vi "Test Classes 2.vi"() -> ()   [LabVIEW 2009]
uses:
  LV-BME Interface/ChnlSettings.ctl
  LV-BME Interface/BME_DG_TriggerSettings.ctl
  LV-BME Interface/ClockSource.ctl
  DG Classes/BME_DG_G08/G08TriggerSettings.ctl
  DG Classes/BME_DG_System/BME_DG_System.lvclass
  DG Classes/BME_DG_G08/BME_DG_G08.lvclass
  DG Classes/BME_DG_G08_Chnl/BME_DG_G08_Chnl.lvclass
  DG Classes/BME_DG_Base/BME_DG_Base.lvclass
  DG Classes/BME_DG_Chnl/BME_DG_Chnl.lvclass
panel:
  in  "Aknowledge interrupts":bool
  in  "stop 3":bool=TRUE
  in  "G08Settings":T1={"Gate Terminate"=TRUE, "Gate Level"=1.0, "Gate Delay (µs)"=0.0, "Step Back Time (µs)"=0.0, "Burst Counter"=0} {"Step Back Time (µs)" min=0.0 format="%.6f"; "Gate Delay (µs)" format="%.3f"; "Gate Level" min=-2.5 max=2.5 format="%.3g"}
  in  "V2 Trigger Settings":T2={"Gate Type"=TRUE, "Synchronize Gate"=FALSE, "Force Trigger (µs)"=0.0, "MS Bus"=1} {"MS Bus" format="%04x" items=["Local Primary"=1, "Local Secondary"=2, "Local Force"=4, "Resynchronize"=8, "Master Primary"=16, "Master Secondary"=32, "Master Force"=64, "System Clock"=128, "Delay Clock"=256, "Inhibit Local"=512, "Start Local"=1024, "Start Bus"=2048, "Step Back Local"=4096, "Step Back Bus"=8192, "Enable From E"=65536, "Enable From F"=131072, "Enable From Bus"=262144]; "Force Trigger (µs)" min=0.0 format="%.6f"}
  in  "SetDelay":bool=TRUE
  in  "UpdateChnl":bool=TRUE
  in  "ChnlParameter":T4 {"ChnParam2write"."Delay (µs)" min=0.0 max=100000000.0 format="%.5f"}
  out "CountsRemains":i32
  out "TriggerCounters":i32[](array[numeric])
  out "Interrupts":u32[](array[numeric]) format="%b"
  in  "ClockSource Master":T5=1 items=["Internal Oscillator"=1, "External Trigger"=2, "Trigger & Oscillator"=3, "MasterSlave Bus"=4]
  in  "Trigger Settings SG02P2":T6={"InputTerminated?"=FALSE, "InternalClockPeriode(µs)"=1000000.0, "TriggerLevel"=1.25, "PresetValue"=0, "DivideBy"=1, "Clock Source"=1, "Gate Divider"=1, "PositiveGate?"=TRUE, "InternalTrigger?"=TRUE, "InternalArm?"=FALSE, "SWTrigger?"=FALSE, "RisingEdge?"=FALSE, "StopOnPreset?"=FALSE, "ResetWhenDone?"=TRUE, "TriggerEnabled?"=TRUE} {"Gate Divider" min=1 max=1000000; "Clock Source" items=["Internal Oscillator"=1, "External Trigger"=2, "Trigger & Oscillator"=3]}
  out "RemainingTriggers":T7(array[cluster])=[[{"Time Stamp"=timestamp(3416308194.6875 s since 1904-01-01), "Numeric"=-64}, {"Time Stamp"=timestamp(3416308194.6875 s since 1904-01-01), "Numeric"=4}, {"Time Stamp"=timestamp(3416308194.6875 s since 1904-01-01), "Numeric"=-64}, {"Time Stamp"=timestamp(3416308194.6875 s since 1904-01-01), "Numeric"=-64}], [{"Time Stamp"=timestamp(3416308194.6875 s since 1904-01-01), "Numeric"=-64}, {"Time Stamp"=timestamp(3416308194.6875 s since 1904-01-01), "Numeric"=-64}, {"Time Stamp"=timestamp(3416308194.6875 s since 1904-01-01), "Numeric"=-64}, {"Time Stamp"=timestamp(3416308194.6875 s since 1904-01-01), "Numeric"=-64}], [{"Time Stamp"=timestamp(3416308194.6875 s since 1904-01-01), "Numeric"=-64}, {"Time Stamp"=timestamp(3416308194.6875 s since 1904-01-01), "Numeric"=-64}, {"Time Stamp"=timestamp(3416308194.6875 s since 1904-01-01), "Numeric"=-64}, {"Time Stamp"=timestamp(3416308194.6875 s since 1904-01-01), "Numeric"=-64}]] {"Time Stamp" format="%<%I:%M:%S%3u %p>T"}
  in  "stop 2":bool=TRUE
  in  "ReadStatus":bool=TRUE
  in  "Activate":bool
  in  "ResetModuloCounters":bool=TRUE
  in  "TriggerModulo":u32=4
  out "Modulo Settings":u32[](array[numeric])
  out "Chnls":T3[](array[typedef])=[{" Delay (µs)"=0.0, "On? (false)"=TRUE, "PositiveVoltage?"=TRUE, "50OhmTerminated? "=TRUE, "25OhmOutput?"=FALSE}, {" Delay (µs)"=0.0, "On? (false)"=TRUE, "PositiveVoltage?"=TRUE, "50OhmTerminated? "=TRUE, "25OhmOutput?"=FALSE}, {" Delay (µs)"=0.0, "On? (false)"=TRUE, "PositiveVoltage?"=TRUE, "50OhmTerminated? "=TRUE, "25OhmOutput?"=FALSE}] {"Delay (µs)" min=0.0 max=100000000.0 format="%.5f"}
  in  "Trigger Base":T6={"InputTerminated?"=FALSE, "InternalClockPeriode(µs)"=1000000.0, "TriggerLevel"=1.25, "PresetValue"=0, "DivideBy"=1, "Clock Source"=1, "Gate Divider"=1, "PositiveGate?"=TRUE, "InternalTrigger?"=FALSE, "InternalArm?"=FALSE, "SWTrigger?"=FALSE, "RisingEdge?"=FALSE, "StopOnPreset?"=FALSE, "ResetWhenDone?"=TRUE, "TriggerEnabled?"=TRUE} {"Gate Divider" min=1 max=1000000; "Clock Source" items=["Internal Oscillator"=1, "External Trigger"=2, "Trigger & Oscillator"=3]}
  in  "Selected Chnl":u16(ring) items=["MasterS08P1_ChnlA", "MasterS08P1_ChnlB", "MasterS08P1_ChnlC", "MasterS08P1_ChnlD", "MasterS08P1_ChnlE", "MasterS08P1_ChnlF"]
  in  "Selected Card":u16(ring)=1 items=["MasterSG02P2", "Slave 1", "Slave 2", "MasterS08P1"]
  in  "STOP":bool=TRUE
  in  "ChnParam2write":T3={" Delay (µs)"=0.0, "On? (false)"=TRUE, "PositiveVoltage?"=TRUE, "50OhmTerminated? "=TRUE, "25OhmOutput?"=FALSE} {"Delay (µs)" min=0.0 max=100000000.0 format="%.5f"}
  # "INIT Values"
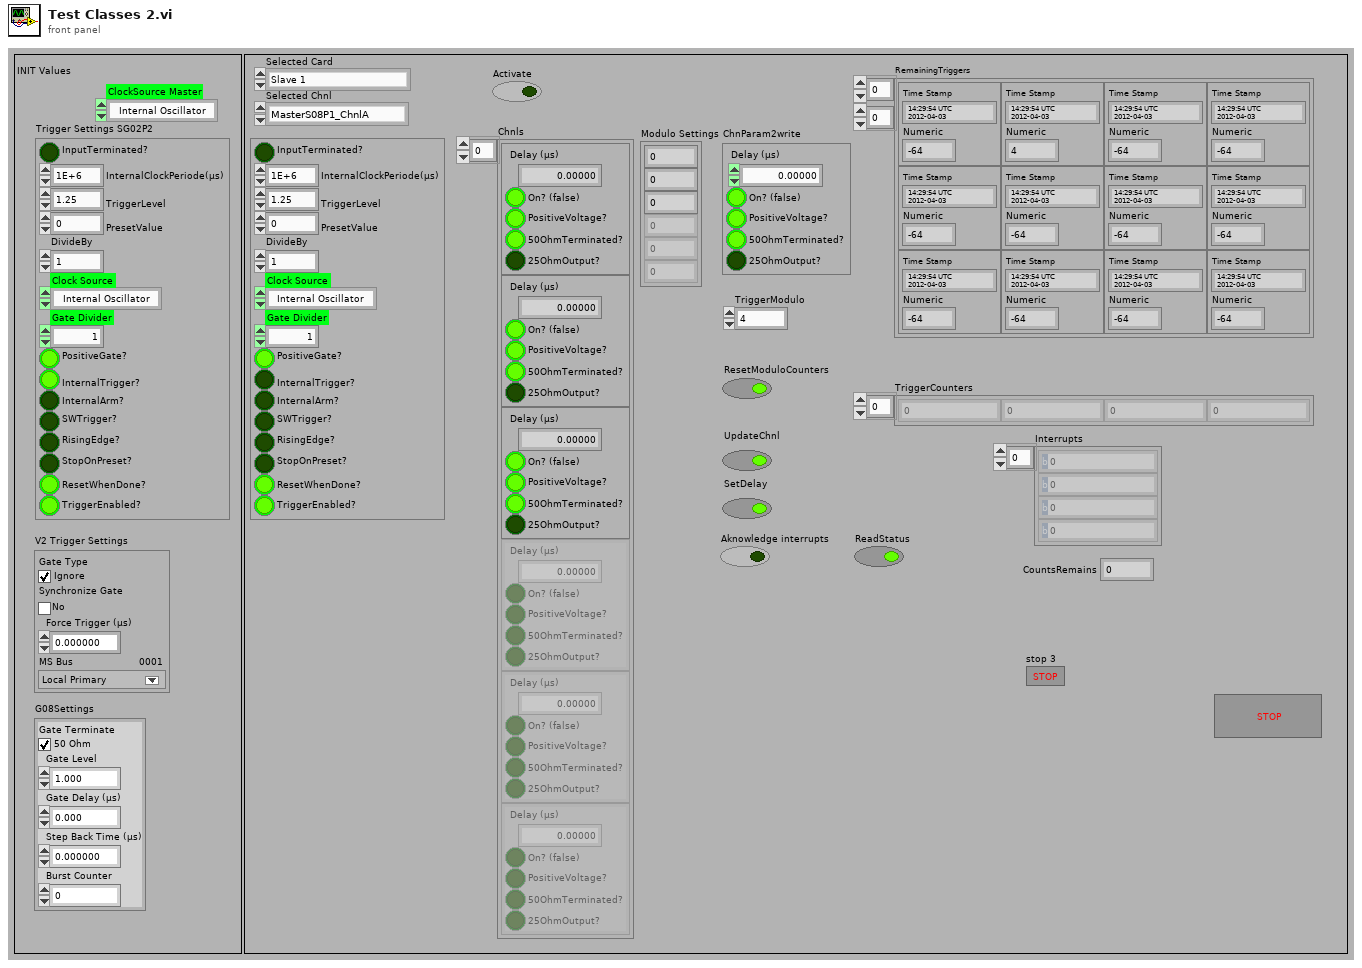
[diagram p1: front panel]
types:
  T1 = typedef "BME_DG_G08.lvclass/G08TriggerSettings.ctl" = cluster{"Gate Terminate":bool, "Gate Level":dbl, "Gate Delay (µs)":dbl, "Step Back Time (µs)":dbl, "Burst Counter":u32}
  T2 = cluster{"Gate Type":bool, "Synchronize Gate":bool, "Force Trigger (µs)":dbl, "MS Bus":u32}
  T3 = typedef "ChnlSettings.ctl" = cluster{" Delay (µs)":dbl, "On? (false)":bool, "PositiveVoltage?":bool, "50OhmTerminated? ":bool, "25OhmOutput?":bool}
  T4 = cluster{"ChnlName":string, "ChnParam2write":T3, "TriggerModulo":u32}
  T5 = typedef "ClockSource.ctl" = i32
  T6 = typedef "BME_DG_TriggerSettings.ctl" = cluster{"InputTerminated?":bool, "InternalClockPeriode(µs)":dbl, "TriggerLevel":dbl, "PresetValue":i32, "DivideBy":i32, "Clock Source":u32, "Gate Divider":i32, "PositiveGate?":bool, "InternalTrigger?":bool, "InternalArm?":bool, "SWTrigger?":bool, "RisingEdge?":bool, "StopOnPreset?":bool, "ResetWhenDone?":bool, "TriggerEnabled?":bool}
  T7 = cluster{"Time Stamp":timestamp, "Numeric":i32}[][]
  T8 = enum8{"Enabled", "Disabled", "Disabled and Grayed Out"}
  T9 = cluster{"ChnlName":string, "ChnParam2write":T3, "TriggerModulo":u32}[]
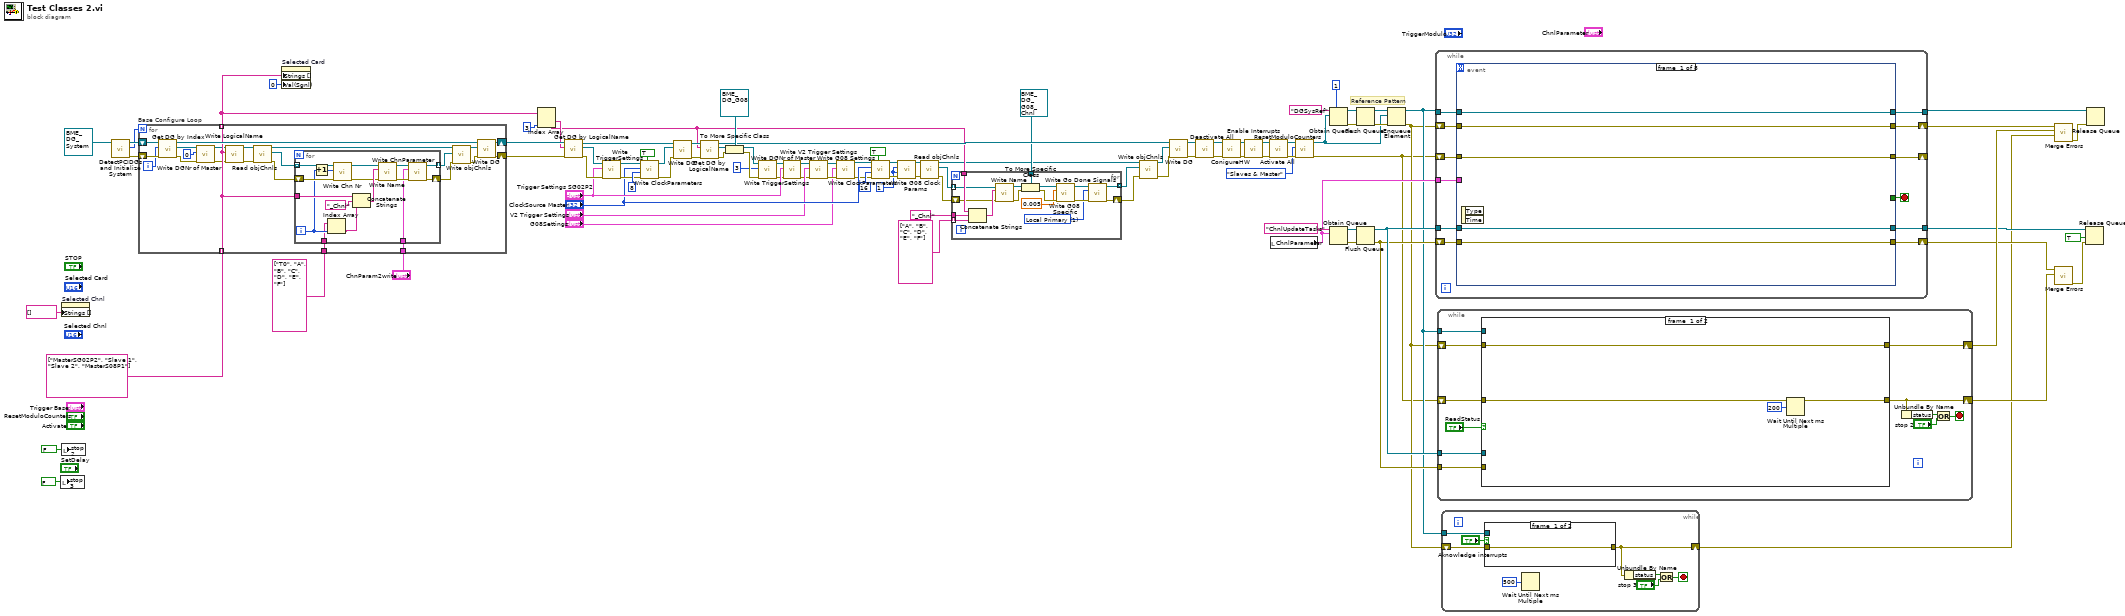
[diagram p0: block diagram]
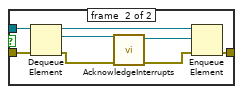
[diagram p2: hidden frame]
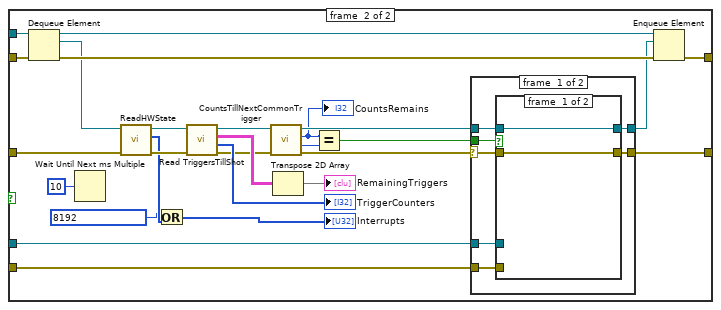
[diagram p3: hidden frame]
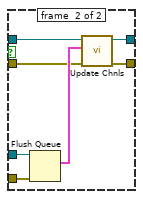
[diagram p4: hidden frame]
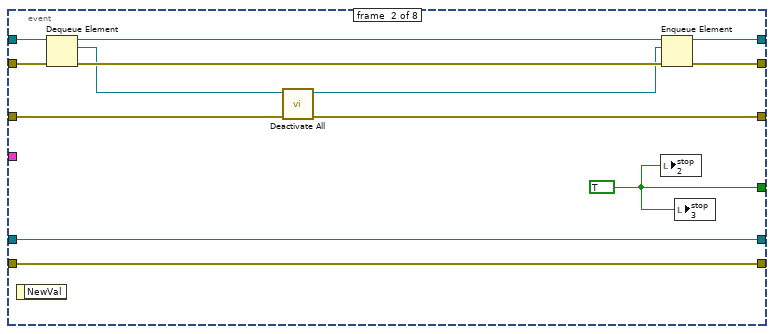
[diagram p6: hidden frame]
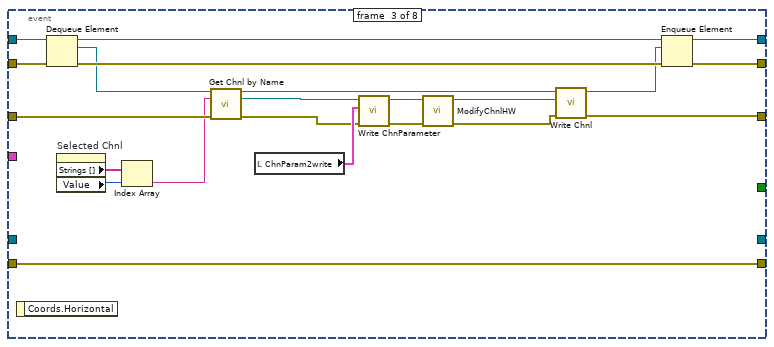
[diagram p7: hidden frame]
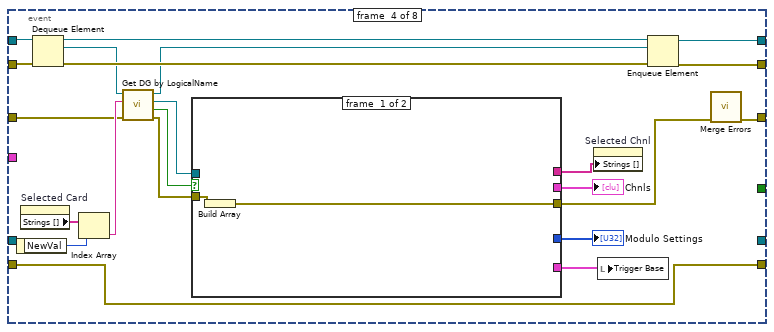
[diagram p8: hidden frame]
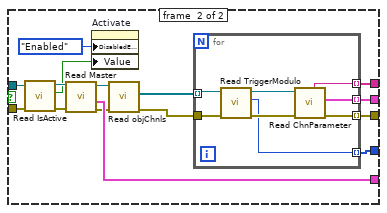
[diagram p9: hidden frame]
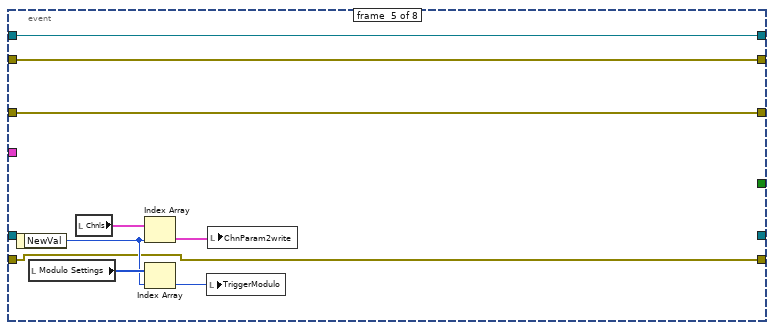
[diagram p10: hidden frame]
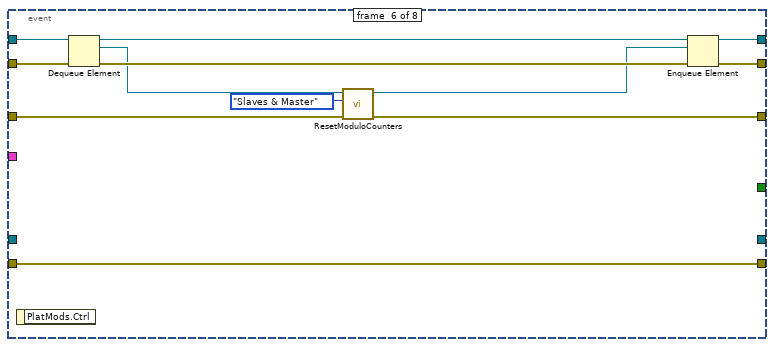
[diagram p11: hidden frame]
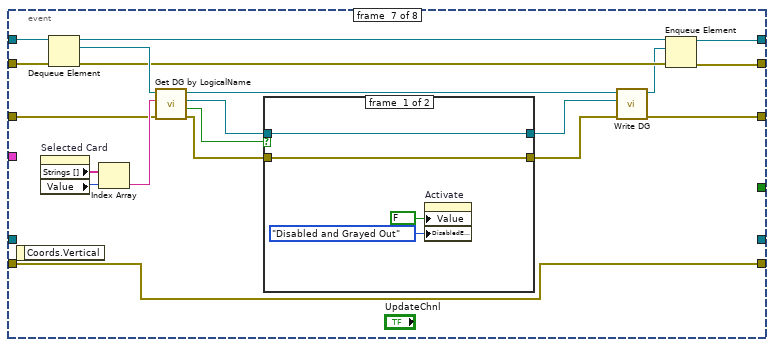
[diagram p12: hidden frame]
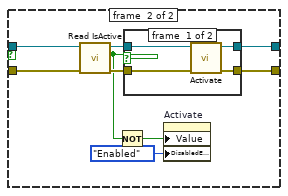
[diagram p13: hidden frame]
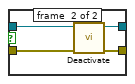
[diagram p14: hidden frame]
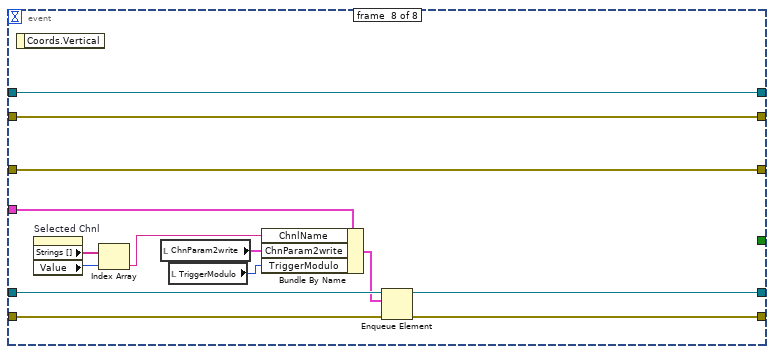
[diagram p15: hidden frame]
diagram:
  w35 = u32 1 ("Trigger Divider")
  # "Reference Pattern"
  n1 = local write "stop 3"(FALSE ("stop 3")) -> ()
  n2 = property on="Selected Chnl" class="Ring (strict)"("Strings []"=string[] []) -> ()  [unwired: 2 in, 2 out]
  n3 = local write "stop 2"(FALSE ("stop 2")) -> ()
  n4 = call "DetectPCIDGs and Initialize System.vi"("BME_DG_System in"=refnum<class "BME_DG_System.lvclass"> refnum ("BME_DG_System.lvclass")) -> ("error out"=w99:errorcluster, "NumberOfCards"=w98:i32, "BME_DG_System out"=w100:refnum<class "BME_DG_System.lvclass">)  [unwired: 8 in]
  n5 = for "Base Configure Loop" {
    N: w98 -> [_]
    shift-right: [w120] -> w68
    shift-left: w100 -> [w124]
    tunnel: string[] ["MasterSG02P2", "Slave 1", "Slave 2", "MasterS08P1"] -> [w109] mode=indexing
    shift-right: [w119] -> w67
    shift-left: w99 -> [w123]
    tunnel: "ChnParam2write" -> [w116]
    tunnel: string[] ["T0", "A", "B", "C", "D", "E", "F"] -> [w110]
    tunnel: [w109] -> w66 mode=indexing
    i -> [w122]
    n6 = call "Get DG by Index.vi"("error in (no error)"=w123, "index"=w122, "BME_DG_System in"=w124) -> ("error out"=w103:errorcluster, "BME_DG_Base.lvclass"=w106:refnum<class "BME_DG_Base.lvclass">, "BME_DG_System out"=w121:refnum<class "BME_DG_System.lvclass">)  [unwired: 6 in]
    n7 = call-dynamic "Write DGNr of Master.vi"("error in (no error)"=w103, "DGNr of Master"=0, "BME_DG_Base in"=w106) -> ("error out"=w104:errorcluster, "BME_DG_Base out"=w105:refnum<class "BME_DG_Base.lvclass">)  [unwired: 7 in]
    n8 = call "Write LogicalName.vi"("error in (no error)"=w104, "LogicalName"=w109, "BME_DG_Base in"=w105) -> ("error out"=w107:errorcluster, "BME_DG_Base out"=w108:refnum<class "BME_DG_Base.lvclass">)  [unwired: 7 in]
    n9 = call-dynamic "Read objChnls.vi"("error in (no error)"=w107, "BME_DG_Base in"=w108) -> ("error out"=w117:errorcluster, "objChnls"=w118:refnum<class "BME_DG_Chnl.lvclass">[], "BME_DG_Base out"=w114:refnum<class "BME_DG_Base.lvclass">)  [unwired: 6 in, 1 out]
    n10 = for {
      tunnel: w118 -> [w134] mode=indexing
      shift-right: [w125] -> w112
      shift-left: w117 -> [w132]
      tunnel: w109 -> [w139]
      tunnel: w116 -> [w135]
      tunnel: [w126] -> w115 mode=indexing
      tunnel: w110 -> [w128]
      i -> [w129]
      n11 = Increment(x=w129) -> (x+1=w130:i32)
      n12 = Index Array(array=w128, index=w129) -> (element=w127:string)
      n13 = call-dynamic "Write Chn Nr.vi"("error in (no error)"=w132, "Chn Nr"=w130, "BME_DG_Chnl in"=w134) -> ("error out"=w131:errorcluster, "BME_DG_Chnl out"=w133:refnum<class "BME_DG_Chnl.lvclass">)  [unwired: 7 in]
      n14 = Concatenate Strings(w139, "_Chnl" ("string"), w127) -> (w137:string)
      n15 = call-dynamic "Write Name.vi"("error in (no error)"=w131, "Name"=w137, "BME_DG_Chnl in"=w133) -> ("error out"=w136:errorcluster, "BME_DG_Chnl out"=w140:refnum<class "BME_DG_Chnl.lvclass">)  [unwired: 7 in]
      n16 = call-dynamic "Write ChnParameter.vi"("error in (no error)"=w136, "ChnParemater"=w135, "BME_DG_Chnl in"=w140) -> ("error out"=w125:errorcluster, "BME_DG_Chnl out"=w126:refnum<class "BME_DG_Chnl.lvclass">)  [unwired: 7 in]
    }
    n17 = call-dynamic "Write objChnls.vi"("error in (no error)"=w112, "objChnls"=w115, "BME_DG_Base in"=w114) -> ("error out"=w111:errorcluster, "BME_DG_Base out"=w113:refnum<class "BME_DG_Base.lvclass">)  [unwired: 7 in]
    n18 = call "Write DG.vi"("error in (no error)"=w111, "BME_DG_Base"=w113, "BME_DG_System in"=w121) -> ("error out"=w119:errorcluster, "BME_DG_System out"=w120:refnum<class "BME_DG_System.lvclass">)  [unwired: 7 in]
  }
  n19 = property on="Selected Card" class="Ring (strict)"("Strings []"=w66, "Val(Sgnl)"=u16 0 ("Value (Signaling)")) -> ()  [unwired: 2 in, 2 out]
  n20 = Index Array(array=w66, index #2=3 ("index")) -> (element #1=w64:string, element #2=w30:string)  [unwired: 1 in]
  n21 = call "Get DG by LogicalName.vi"("error in (no error)"=w67, "LogicalName"=w64, "BME_DG_System in"=w68) -> ("error out"=w62:errorcluster, "BME_DG_Base.lvclass"=w63:refnum<class "BME_DG_Base.lvclass">, "BME_DG_System out"=w59:refnum<class "BME_DG_System.lvclass">)  [unwired: 5 in, 1 out]
  n22 = call-dynamic "Write TriggerSettings.vi"("error in (no error)"=w62, "Trigger Settings"="Trigger Settings SG02P2", "BME_DG_Base in"=w63) -> ("error out"=w60:errorcluster, "BME_DG_Base out"=w61:refnum<class "BME_DG_Base.lvclass">)  [unwired: 7 in]
  n23 = call-dynamic "Write ClockParameters.vi"("ClockEnable"=TRUE, "error in (no error)"=w60, "PrescalerCrystalOscilator"=u32 8 ("DivideBy"), "ClockSource"="ClockSource Master", "BME_DG_Base in"=w61) -> ("error out"=w57:errorcluster, "BME_DG_Base out"=w58:refnum<class "BME_DG_Base.lvclass">)  [unwired: 5 in]
  n24 = call "Write DG.vi"("error in (no error)"=w57, "BME_DG_Base"=w58, "BME_DG_System in"=w59) -> ("error out"=w56:errorcluster, "BME_DG_System out"=w55:refnum<class "BME_DG_System.lvclass">)  [unwired: 7 in]
  n25 = call "Get DG by LogicalName.vi"("error in (no error)"=w56, "LogicalName"=w30, "BME_DG_System in"=w55) -> ("error out"=w45:errorcluster, "BME_DG_Base.lvclass"=w50:refnum<class "BME_DG_Base.lvclass">, "BME_DG_System out"=w41:refnum<class "BME_DG_System.lvclass">)  [unwired: 5 in, 1 out]
  n26 = To More Specific Class(target class=refnum<class "BME_DG_G08.lvclass"> refnum ("BME_DG_G08.lvclass"), reference=w50, error in=w45) -> (specific class reference=w16:refnum<class "BME_DG_G08.lvclass">, error out=w14:errorcluster)
  n27 = call-dynamic "Write DGNr of Master.vi"("error in (no error)"=w14, "DGNr of Master"=3, "BME_DG_Base in"=w16) -> ("error out"=w13:errorcluster, "BME_DG_Base out"=w15:refnum<class "BME_DG_G08.lvclass">)  [unwired: 7 in]
  n28 = call-dynamic "Write TriggerSettings.vi"("error in (no error)"=w13, "Trigger Settings"="Trigger Settings SG02P2", "BME_DG_Base in"=w15) -> ("error out"=w46:errorcluster, "BME_DG_Base out"=w48:refnum<class "BME_DG_G08.lvclass">)  [unwired: 7 in]
  n29 = call-dynamic "Write V2 Trigger Settings.vi"("error in (no error)"=w46, "V2 Trigger Settings"="V2 Trigger Settings", "BME_DG_G05 in"=w48) -> ("error out"=w43:errorcluster, "BME_DG_G05 out"=w44:refnum<class "BME_DG_G08.lvclass">)  [unwired: 7 in]
  n30 = call-dynamic "Write G08 Settings.vi"("error in (no error)"=w43, "G08Settings"="G08Settings", "BME_DG_G08 in"=w44) -> ("error out"=w38:errorcluster, "BME_DG_G08 out"=w39:refnum<class "BME_DG_G08.lvclass">)  [unwired: 7 in]
  n31 = call-dynamic "Write ClockParameters.vi"("ClockEnable"=TRUE, "error in (no error)"=w38, "PrescalerCrystalOscilator"=u32 16, "ClockSource"="ClockSource Master", "BME_DG_Base in"=w39) -> ("error out"=w36:errorcluster, "BME_DG_Base out"=w37:refnum<class "BME_DG_G08.lvclass">)  [unwired: 5 in]
  n32 = call-dynamic "Write G08 Clock Params.vi"("error in (no error)"=w36, "Trigger Multiplier"=w35, "Trigger Divider"=w35, "BME_DG_G08 in"=w37) -> ("error out"=w33:errorcluster, "BME_DG_G08 out"=w34:refnum<class "BME_DG_G08.lvclass">)  [unwired: 6 in]
  n33 = call-dynamic "Read objChnls.vi"("error in (no error)"=w33, "BME_DG_Base in"=w34) -> ("error out"=w29:errorcluster, "objChnls"=w32:refnum<class "BME_DG_Chnl.lvclass">[], "BME_DG_Base out"=w25:refnum<class "BME_DG_G08.lvclass">)  [unwired: 6 in, 1 out]
  n34 = for {
    tunnel: w32 -> [w155] mode=indexing
    tunnel: string[] ["A", "B", "C", "D", "E", "F"] -> [w157] mode=indexing
    tunnel: w30 -> [w156]
    shift-right: [w144] -> w26
    shift-left: w29 -> [w153]
    tunnel: "_Chnl" ("string") -> [w152]
    tunnel: refnum<class "BME_DG_G08_Chnl.lvclass"> refnum ("BME_DG_G08_Chnl.lvclass") -> [w149]
    tunnel: [w142] -> w24 mode=indexing
    w143 = u32 1 items=["Local Primary"=1, "Local Secondary"=2, "Local Force"=4, "Resynchronize"=8, "Master Primary"=16, "Master Secondary"=32, "Master Force"=64, "System Clock"=128, "Delay Clock"=256, "Inhibit Local"=512, "Start Local"=1024, "Start Bus"=2048, "Step Back Local"=4096, "Step Back Bus"=8192, "From E"=65536, "From F"=131072, "From Bus"=262144] ("Go Signal")
    n35 = Concatenate Strings(w156, w152, w157) -> (w154:string)
    n36 = call-dynamic "Write Name.vi"("error in (no error)"=w153, "Name"=w154, "BME_DG_Chnl in"=w155) -> ("error out"=w148:errorcluster, "BME_DG_Chnl out"=w151:refnum<class "BME_DG_Chnl.lvclass">)  [unwired: 7 in]
    n37 = To More Specific Class(target class=w149, reference=w151, error in=w148) -> (specific class reference=w150:refnum<class "BME_DG_G08_Chnl.lvclass">, error out=w147:errorcluster)
    n38 = call-dynamic "Write G08 Specific.vi"("error in (no error)"=w147, "Pulse Width (µs)"=0.005, "BME_DG_G08_Chnl in"=w150) -> ("error out"=w145:errorcluster, "BME_DG_G08_Chnl out"=w146:refnum<class "BME_DG_G08_Chnl.lvclass">)  [unwired: 7 in]
    n39 = call-dynamic "Write Go Done Signals.vi"("error in (no error)"=w145, "Go Signal"=w143, "BME_DG_G05P2_Chnl in"=w146) -> ("error out"=w144:errorcluster, "BME_DG_G05P2_Chnl out"=w142:refnum<class "BME_DG_G08_Chnl.lvclass">)  [unwired: 7 in]
  }
  n40 = call-dynamic "Write objChnls.vi"("error in (no error)"=w26, "objChnls"=w24, "BME_DG_Base in"=w25) -> ("error out"=w22:errorcluster, "BME_DG_Base out"=w23:refnum<class "BME_DG_G08.lvclass">)  [unwired: 7 in]
  n41 = call "Write DG.vi"("error in (no error)"=w22, "BME_DG_Base"=w23, "BME_DG_System in"=w41) -> ("error out"=w21:errorcluster, "BME_DG_System out"=w40:refnum<class "BME_DG_System.lvclass">)  [unwired: 7 in]
  n42 = call "Deactivate All.vi"("error in (no error)"=w21, "BME_DG_System in"=w40) -> ("error out"=w19:errorcluster, "BME_DG_System out"=w20:refnum<class "BME_DG_System.lvclass">)  [unwired: 8 in]
  n43 = call "ConigureHW.vi"("error in (no error)"=w19, "BME_DG_System in"=w20) -> ("error out"=w17:errorcluster, "BME_DG_System out"=w18:refnum<class "BME_DG_System.lvclass">)  [unwired: 8 in]
  n44 = call "Enable Interrupts.vi"("error in (no error)"=w17, "BME_DG_System in"=w18) -> ("error out"=w6:errorcluster, "BME_DG_System out"=w7:refnum<class "BME_DG_System.lvclass">)  [unwired: 8 in]
  n45 = call "Activate All.vi"("error in (no error)"=w6, "BME_DG_System in"=w7) -> ("error out"=w3:errorcluster, "BME_DG_System out"=w5:refnum<class "BME_DG_System.lvclass">)  [unwired: 8 in]
  n46 = local read "ChnlParameter"() -> (w78:T4)
  n47 = call "ResetModuloCounters.vi"("error in (no error)"=w3, "Enum"=enum16{"Slaves only", "Slaves & Master"}."Slaves & Master", "BME_DG_System in"=w5) -> ("error out"=w2:errorcluster, "BME_DG_System out"=w4:refnum<class "BME_DG_System.lvclass">)  [unwired: 7 in]
  n48 = Obtain Queue(max queue size (-1, unlimited)=1, name (unnamed)="DGSysRef", element data type=w4) -> (queue out=w86:refnum<queue>, error out=w84:errorcluster)  [unwired: 2 in, 1 out]
  n49 = Obtain Queue(name (unnamed)="ChnlUpdateTasks", element data type=w78) -> (queue out=w79:refnum<queue>, error out=w80:errorcluster)  [unwired: 3 in, 1 out]
  n50 = Flush Queue(queue=w86, error in (no error)=w84) -> (queue out=w85:refnum<queue>, error out=w83:errorcluster)  [unwired: 1 out]
  n51 = Flush Queue(queue=w79, error in (no error)=w80) -> (queue out=w75:refnum<queue>, error out=w74:errorcluster)  [unwired: 1 out]
  n52 = Enqueue Element(queue=w85, element=w4, error in (no error)=w83) -> (queue out=w11:refnum<queue>, error out=w10:errorcluster)  [unwired: 1 in, 1 out]
  n53 = while {
    shift-right: [w165] -> _
    shift-left: w2 -> [w167]
    shift-right: [w163] -> w89
    shift-left: w10 -> [w164]
    tunnel: w11 -> [w168]
    tunnel: [w166] -> w91
    tunnel: w75 -> [w162]
    tunnel: w78 -> [w161]
    tunnel: [w159] -> w77
    shift-right: [w158] -> w73
    shift-left: w74 -> [w160]
    stop <- w169 stop-if-true
    n54 = event shown="[1] \"STOP\": Value Change" {
      selector: _ -> [_ _ _ _ _ _ _ _]
      dyn-events: _ -> [_ _ _ _ _ _ _ _]
      timeout: _ -> [_ _ _ _ _ _ _ _]
      tunnel: [_ w175 _ _ _ _ _ _] -> w169
      tunnel: w168 -> [w174 w184 w208 w219 w265 w277 w286 w332]
      tunnel: w167 -> [w173 w187 w199 w228 w264 w267 w294 w331]
      tunnel: [w174 w180 w204 w217 w265 w272 w280 w332] -> w166
      tunnel: [w173 w186 w188 w212 w264 w268 w287 w331] -> w165
      tunnel: w164 -> [w172 w183 w207 w218 w258 w275 w285 w328]
      tunnel: [w172 w181 w205 w216 w258 w273 w279 w328] -> w163
      tunnel: w162 -> [w171 w177 _ _ _ _ _ w323]
      tunnel: w161 -> [_ _ _ _ _ _ _ w327]
      tunnel: w160 -> [w170 w176 w203 w210 w257 w271 w278 w321]
      tunnel: [w171 w177 _ _ _ _ _ w320] -> w159
      tunnel: [w170 w176 w203 w210 w257 w271 w278 w319] -> w158
      event #0 {
        n55 = event-data() -> ()  [unwired: 1 in, 2 out]
      }
      event #1 {
        w175 = TRUE
        n56 = event-data() -> ()  [unwired: 1 in, 1 out]
        n57 = Dequeue Element(queue=w184, error in (no error)=w183) -> (queue out=w185:refnum<queue>, element=w178:refnum<class "BME_DG_System.lvclass">, error out=w182:errorcluster)  [unwired: 1 in, 1 out]
        n58 = call "Deactivate All.vi"("error in (no error)"=w187, "BME_DG_System in"=w178) -> ("error out"=w186:errorcluster, "BME_DG_System out"=w179:refnum<class "BME_DG_System.lvclass">)  [unwired: 8 in]
        n59 = local write "stop 2"(w175) -> ()
        n60 = Enqueue Element(queue=w185, element=w179, error in (no error)=w182) -> (queue out=w180:refnum<queue>, error out=w181:errorcluster)  [unwired: 1 in, 1 out]
        n61 = local write "stop 3"(w175) -> ()
      }
      event #2 {
        n62 = event-data() -> ()  [unwired: 1 in, 1 out]
        n63 = Dequeue Element(queue=w208, error in (no error)=w207) -> (queue out=w209:refnum<queue>, element=w200:refnum<class "BME_DG_System.lvclass">, error out=w206:errorcluster)  [unwired: 1 in, 1 out]
        n64 = property on="Selected Chnl" class="Ring (strict)"() -> ("Strings []"=w201:string[], "Value"=w202:u16)  [unwired: 2 in, 2 out]
        n65 = Index Array(array=w201, index=w202) -> (element=w198:string)
        n66 = call "Get Chnl by Name.vi"("BME_DG_System in"=w200, "Chnl Name"=w198, "error in (no error)"=w199) -> ("BME_DG_System out"=w194:refnum<class "BME_DG_System.lvclass">, "BME_DG_Chnl"=w197:refnum<class "BME_DG_Chnl.lvclass">, "error out"=w195:errorcluster)  [unwired: 7 in, 3 out]
        n67 = local read "ChnParam2write"() -> (w196:T3)
        n68 = call-dynamic "Write ChnParameter.vi"("error in (no error)"=w195, "ChnParemater"=w196, "BME_DG_Chnl in"=w197) -> ("error out"=w191:errorcluster, "BME_DG_Chnl out"=w192:refnum<class "BME_DG_Chnl.lvclass">)  [unwired: 7 in]
        n69 = call-dynamic "ModifyChnlHW.vi"("error in (no error)"=w191, "BME_DG_Chnl in"=w192) -> ("error out"=w189:errorcluster, "BME_DG_Chnl out"=w190:refnum<class "BME_DG_Chnl.lvclass">)  [unwired: 8 in]
        n70 = call "Write Chnl.vi"("error in (no error)"=w189, "BME_DG_Chnl.lvclass"=w190, "BME_DG_System in"=w194) -> ("error out"=w188:errorcluster, "BME_DG_System out"=w193:refnum<class "BME_DG_System.lvclass">)  [unwired: 7 in]
        n71 = Enqueue Element(queue=w209, element=w193, error in (no error)=w206) -> (queue out=w204:refnum<queue>, error out=w205:errorcluster)  [unwired: 1 in, 1 out]
      }
      event #3 {
        n72 = event-data() -> ("NewVal"=w230:u16)  [unwired: 1 in]
        n73 = property on="Selected Card" class="Ring (strict)"() -> ("Strings []"=w231:string[])  [unwired: 2 in, 2 out]
        n74 = Dequeue Element(queue=w219, error in (no error)=w218) -> (queue out=w220:refnum<queue>, element=w215:refnum<class "BME_DG_System.lvclass">, error out=w221:errorcluster)  [unwired: 1 in, 1 out]
        n75 = Index Array(array=w231, index=w230) -> (element=w229:string)
        n76 = call "Get DG by LogicalName.vi"("error in (no error)"=w228, "LogicalName"=w229, "BME_DG_System in"=w215) -> ("error out"=w213:errorcluster, "found?"=w227:bool, "BME_DG_Base.lvclass"=w226:refnum<class "BME_DG_Base.lvclass">, "BME_DG_System out"=w214:refnum<class "BME_DG_System.lvclass">)  [unwired: 5 in]
        n77 = case shown="True" w227 {
          tunnel: w226 -> [_ w241]
          tunnel: [_ w248] -> w225
          tunnel: [_ w247] -> w223
          tunnel: [_ w246] -> w224
          tunnel: [_ w242] -> w222
          tunnel: w213 -> [w233 w238]
          tunnel: [w232 w236] -> w211
          frame #0 {
            n78 = Build Array(w233) -> (w232:errorcluster[])
          }
          frame #1 {
            n79 = call-dynamic "Read IsActive.vi"("error in (no error)"=w238, "BME_DG_Base in"=w241) -> ("error out"=w239:errorcluster, "Active?"=w234:bool, "BME_DG_Base out"=w240:refnum<class "BME_DG_Base.lvclass">)  [unwired: 7 in]
            n80 = call-dynamic "Read Master.vi"("error in (no error)"=w239, "BME_DG_Base in"=w240) -> ("error out"=w243:errorcluster, "TriggerSettings"=w246:T6, "BME_DG_Base out"=w244:refnum<class "BME_DG_Base.lvclass">)  [unwired: 6 in, 1 out]
            n81 = property on="Activate" class="Bool (strict)"("DisabledEnum"=T8."Enabled" ("Disabled"), "Value"=w234) -> ()  [unwired: 2 in, 2 out]
            n82 = call-dynamic "Read objChnls.vi"("error in (no error)"=w243, "BME_DG_Base in"=w244) -> ("error out"=w237:errorcluster, "objChnls"=w245:refnum<class "BME_DG_Chnl.lvclass">[])  [unwired: 6 in, 2 out]
            n83 = for {
              tunnel: w245 -> [w254] mode=indexing
              tunnel: [w256] -> w248 mode=indexing
              tunnel: [w255] -> w247 mode=indexing
              tunnel: [w249] -> w242 mode=indexing
              tunnel: w237 -> [w252]
              tunnel: [w250] -> w236 mode=indexing
              n84 = call-dynamic "Read TriggerModulo.vi"("error in (no error)"=w252, "BME_DG_Chnl in"=w254) -> ("error out"=w251:errorcluster, "TriggerModulo"=w249:i32, "BME_DG_Chnl out"=w253:refnum<class "BME_DG_Chnl.lvclass">)  [unwired: 7 in]
              n85 = call-dynamic "Read ChnParameter.vi"("error in (no error)"=w251, "BME_DG_Chnl in"=w253) -> ("error out"=w250:errorcluster, "ChnParemater"=w255:T3, "Name"=w256:string)  [unwired: 4 in, 3 out]
            }
          }
        }
        "Chnls" <- w223
        "Modulo Settings" <- w222
        n86 = property on="Selected Chnl" class="Ring (strict)"("Strings []"=w225) -> ()  [unwired: 2 in, 2 out]
        n87 = local write "Trigger Base"(w224) -> ()
        n88 = Enqueue Element(queue=w220, element=w214, error in (no error)=w221) -> (queue out=w217:refnum<queue>, error out=w216:errorcluster)  [unwired: 1 in, 1 out]
        n89 = call <vilib>:"Merge Errors.vi"("error array in"=w211) -> ("error out"=w212:errorcluster)  [unwired: 6 in]
      }
      event #4 {
        n90 = event-data() -> ("NewVal"=w261:u16)  [unwired: 1 in]
        n91 = local read "Modulo Settings"() -> (w262:u32[])
        n92 = local read "Chnls"() -> (w263:T3[])
        n93 = Index Array(array=w263, index=w261) -> (element=w260:T3)
        n94 = Index Array(array=w262, index=w261) -> (element=w259:u32)
        n95 = local write "TriggerModulo"(w259) -> ()
        n96 = local write "ChnParam2write"(w260) -> ()
      }
      event #5 {
        n97 = event-data() -> ()  [unwired: 1 in, 1 out]
        n98 = Dequeue Element(queue=w277, error in (no error)=w275) -> (queue out=w276:refnum<queue>, element=w270:refnum<class "BME_DG_System.lvclass">, error out=w274:errorcluster)  [unwired: 1 in, 1 out]
        n99 = call "ResetModuloCounters.vi"("error in (no error)"=w267, "Enum"=enum16{"Slaves only", "Slaves & Master"}."Slaves & Master", "BME_DG_System in"=w270) -> ("error out"=w268:errorcluster, "BME_DG_System out"=w269:refnum<class "BME_DG_System.lvclass">)  [unwired: 7 in]
        n100 = Enqueue Element(queue=w276, element=w269, error in (no error)=w274) -> (queue out=w272:refnum<queue>, error out=w273:errorcluster)  [unwired: 1 in, 1 out]
      }
      event #6 {
        n101 = event-data() -> ()  [unwired: 1 in, 1 out]
        n102 = property on="Selected Card" class="Ring (strict)"() -> ("Strings []"=w297:string[], "Value"=w296:u16)  [unwired: 2 in, 2 out]
        n103 = Dequeue Element(queue=w286, error in (no error)=w285) -> (queue out=w283:refnum<queue>, element=w284:refnum<class "BME_DG_System.lvclass">, error out=w282:errorcluster)  [unwired: 1 in, 1 out]
        n104 = Index Array(array=w297, index=w296) -> (element=w295:string)
        n105 = call "Get DG by LogicalName.vi"("error in (no error)"=w294, "LogicalName"=w295, "BME_DG_System in"=w284) -> ("error out"=w292:errorcluster, "found?"=w288:bool, "BME_DG_Base.lvclass"=w293:refnum<class "BME_DG_Base.lvclass">, "BME_DG_System out"=w289:refnum<class "BME_DG_System.lvclass">)  [unwired: 5 in]
        n106 = case shown="True" w288 {
          tunnel: w293 -> [w301 w308]
          tunnel: w292 -> [w300 w306]
          tunnel: [w300 w310] -> w291
          tunnel: [w301 w309] -> w290
          frame #0 {
            n107 = property on="Activate" class="Bool (strict)"("Value"=FALSE ("Activate"), "DisabledEnum"=T8."Disabled and Grayed Out" ("Disabled")) -> ()  [unwired: 2 in, 2 out]
          }
          frame #1 {
            n108 = call-dynamic "Read IsActive.vi"("error in (no error)"=w306, "BME_DG_Base in"=w308) -> ("error out"=w305:errorcluster, "Active?"=w304:bool, "BME_DG_Base out"=w307:refnum<class "BME_DG_Base.lvclass">)  [unwired: 7 in]
            n109 = Not(x=w304) -> (.not. x?=w302:bool)
            n110 = case shown="True" w304 {
              tunnel: [w314 w316] -> w310
              tunnel: [w313 w317] -> w309
              tunnel: w307 -> [w312 w318]
              tunnel: w305 -> [w311 w315]
              frame #0 {
                n111 = call-dynamic "Activate.vi"("error in (no error)"=w311, "BME_DG_Base in"=w312) -> ("error out"=w314:errorcluster, "BME_DG_Base out"=w313:refnum<class "BME_DG_Base.lvclass">)  [unwired: 8 in]
              }
              frame #1 {
                n112 = call-dynamic "Deactivate.vi"("error in (no error)"=w315, "BME_DG_Base in"=w318) -> ("error out"=w316:errorcluster, "BME_DG_Base out"=w317:refnum<class "BME_DG_Base.lvclass">)  [unwired: 8 in]
              }
            }
            n113 = property on="Activate" class="Bool (strict)"("Value"=w302, "DisabledEnum"=T8."Enabled" ("Disabled")) -> ()  [unwired: 2 in, 2 out]
          }
        }
        n114 = call "Write DG.vi"("error in (no error)"=w291, "BME_DG_Base"=w290, "BME_DG_System in"=w289) -> ("error out"=w287:errorcluster, "BME_DG_System out"=w281:refnum<class "BME_DG_System.lvclass">)  [unwired: 7 in]
        n115 = Enqueue Element(queue=w283, element=w281, error in (no error)=w282) -> (queue out=w280:refnum<queue>, error out=w279:errorcluster)  [unwired: 1 in, 1 out]
      }
      event #7 {
        n116 = event-data() -> ()  [unwired: 1 in, 1 out]
        n117 = property on="Selected Chnl" class="Ring (strict)"() -> ("Strings []"=w329:string[], "Value"=w330:u16)  [unwired: 2 in, 2 out]
        n118 = Index Array(array=w329, index=w330) -> (element=w326:string)
        n119 = local read "ChnParam2write"() -> (w325:T3)
        n120 = local read "TriggerModulo"() -> (w324:u32)
        n121 = Bundle By Name(cluster=w327, "ChnlName"=w326, "ChnParam2write"=w325, "TriggerModulo"=w324) -> (w322:T4)
        n122 = Enqueue Element(queue=w323, element=w322, error in (no error)=w321) -> (queue out=w320:refnum<queue>, error out=w319:errorcluster)  [unwired: 1 in, 1 out]
      }
    }
  }
  n123 = while {
    tunnel: w11 -> [w340]
    shift-right: [w338] -> w88
    shift-left: w10 -> [w339]
    shift-right: [w335] -> w72
    shift-left: w2 -> [w337]
    tunnel: w75 -> [w334]
    tunnel: w74 -> [w333]
    stop <- w342 stop-if-true
    n124 = case shown="True" "ReadStatus" {
      tunnel: w340 -> [_ w371]
      tunnel: w339 -> [w345 w370]
      tunnel: [w345 w369] -> w338
      tunnel: w337 -> [w344 w367]
      tunnel: [w344 w353] -> w335
      tunnel: w334 -> [_ w357]
      tunnel: w333 -> [_ w356]
      frame #0 {
        n125 = Wait Until Next ms Multiple(millisecond multiple=u32 200) -> ()  [unwired: 1 out]
      }
      frame #1 {
        n126 = Dequeue Element(queue=w371, error in (no error)=w370) -> (queue out=w372:refnum<queue>, element=w368:refnum<class "BME_DG_System.lvclass">, error out=w373:errorcluster)  [unwired: 1 in, 1 out]
        n127 = Wait Until Next ms Multiple(millisecond multiple=u32 10) -> ()  [unwired: 1 out]
        n128 = call "ReadHWState.vi"("error in (no error)"=w367, "BME_DG_System in"=w368) -> ("error out"=w366:errorcluster, "Interrupts"=w362:u32[], "BME_DG_System out"=w365:refnum<class "BME_DG_System.lvclass">)  [unwired: 7 in]
        n129 = Or(x=u32 8192, y=w362) -> (x .or. y?=→"Interrupts":u32[])
        n130 = call "Read TriggersTillShot.vi"("error in (no error)"=w366, "BME_DG_System in"=w365) -> ("error out"=w358:errorcluster, "TriggerCounters"=→"TriggerCounters":i32[], "RemainingTriggers"=w364:T7, "BME_DG_System out"=w359:refnum<class "BME_DG_System.lvclass">)  [unwired: 6 in]
        n131 = call "CountsTillNextCommonTrigger.vi"("error in (no error)"=w358, "BME_DG_System in"=w359) -> ("error out"=w355:errorcluster, "LeastCommonMult"=w350:i32, "CountsRemains"=w351:i32, "BME_DG_System out"=w354:refnum<class "BME_DG_System.lvclass">)  [unwired: 6 in]
        "CountsRemains" <- w351
        n132 = Transpose 2D Array(2D array=w364) -> (transposed array=→"RemainingTriggers":T7)
        n133 = Equal?(x=w351, y=w350) -> (x = y?=w349:bool)
        n134 = case shown="No Error" w355 {
          selector: w355 -> [w377 w390]
          tunnel: w357 -> [w380 _]
          tunnel: w356 -> [w379 _]
          tunnel: w354 -> [w378 w391]
          tunnel: [w376 w390] -> w353
          tunnel: [w375 w391] -> w352
          tunnel: w349 -> [w374 _]
          frame #0 {
            n135 = case shown="True" w374 {
              tunnel: w380 -> [_ w389]
              tunnel: w379 -> [_ w388]
              tunnel: w378 -> [w382 w387]
              tunnel: w377 -> [w381 w385]
              tunnel: [w381 w384] -> w376
              tunnel: [w382 w383] -> w375
              frame #0 {
              }
              frame #1 {
                n136 = Flush Queue(queue=w389, error in (no error)=w388) -> (remaining elements=w386:T9)  [unwired: 2 out]
                n137 = call "Update Chnls.vi"("error in (no error)"=w385, "ChnlSettings"=w386, "BME_DG_System in"=w387) -> ("error out"=w384:errorcluster, "BME_DG_System out"=w383:refnum<class "BME_DG_System.lvclass">)  [unwired: 7 in]
              }
            }
          }
          frame #1 {
          }
        }
        n138 = Enqueue Element(queue=w372, element=w352, error in (no error)=w373) -> (error out=w369:errorcluster)  [unwired: 1 in, 2 out]
      }
    }
    n139 = Unbundle By Name(w335) -> ("status"=w341:bool)
    n140 = Or(x=w341, y="stop 2") -> (x .or. y?=w342:bool)
  }
  n141 = while {
    tunnel: w11 -> [w396]
    shift-right: [w393] -> w8
    shift-left: w10 -> [w395]
    stop <- w398 stop-if-true
    n142 = case shown="True" "Aknowledge interrupts" {
      tunnel: w396 -> [_ w408]
      tunnel: w395 -> [w400 w407]
      tunnel: [w400 w406] -> w393
      frame #0 {
      }
      frame #1 {
        n143 = Dequeue Element(queue=w408, error in (no error)=w407) -> (queue out=w405:refnum<queue>, element=w404:refnum<class "BME_DG_System.lvclass">, error out=w403:errorcluster)  [unwired: 1 in, 1 out]
        n144 = call "AcknowledgeInterrupts.vi"("error in (no error)"=w403, "BME_DG_System in"=w404) -> ("error out"=w401:errorcluster, "BME_DG_System out"=w402:refnum<class "BME_DG_System.lvclass">)  [unwired: 8 in]
        n145 = Enqueue Element(queue=w405, element=w402, error in (no error)=w401) -> (error out=w406:errorcluster)  [unwired: 1 in, 2 out]
      }
    }
    n146 = Wait Until Next ms Multiple(millisecond multiple=u32 500) -> ()  [unwired: 1 out]
    n147 = Unbundle By Name(w393) -> ("status"=w397:bool)
    n148 = Or(x=w397, y="stop 3") -> (x .or. y?=w398:bool)
  }
  n149 = call <vilib>:"Merge Errors.vi"("error in 3 (no error)"=w8, "error in 2 (no error)"=w88, "error in 1 (no error)"=w89) -> ("error out"=w90:errorcluster)  [unwired: 4 in]
  n150 = call <vilib>:"Merge Errors.vi"("error in 2 (no error)"=w72, "error in 1 (no error)"=w73) -> ("error out"=w71:errorcluster)  [unwired: 5 in]
  n151 = Release Queue(queue=w77, force destroy? (F)=TRUE, error in (no error)=w71) -> ()  [unwired: 3 out]
  n152 = Release Queue(queue=w91, error in (no error)=w90) -> ()  [unwired: 1 in, 3 out]
